vi "motors.vi"() -> (13 "Faults":bool[](array[boolean]), 14 "Left Drive 1":bool, 15 "Left Drive 2":bool, 16 "Left Drive 3":bool, 17 "Right Drive 1":bool, 18 "Right Drive 2":bool, 19 "Right Drive 3":bool)   [LabVIEW 2015]
uses:
  <vilib>/Rock Robotics/Network Tables/NT Read Number.vi
panel:
  out "Right Talon 1 Temperature Fault":i32
  out "Right Talon 1 Voltage Fault":i32
  out "Right Talon 1 Hardware Fault":i32
  out "Right Talon 2 Temperature Fault":i32
  out "Right Talon 2 Voltage Fault":i32
  out "Right Talon 2 Hardware Fault":i32
  out "Right Talon 3 Temperature Fault":i32
  out "Right Talon 3 Voltage Fault":i32
  out "Right Talon 3 Hardware Fault":i32
  out "Left Talon 3 Temperature Fault":i32
  out "Left Talon 3 Voltage Fault":i32
  out "Left Talon 3 Hardware Fault":i32
  out "Left Talon 2 Temperature Fault":i32
  out "Left Talon 2 Voltage Fault":i32
  out "Left Talon 2 Hardware Fault":i32
  out "Left Talon 1 Hardware Fault":i32
  out "Left Talon 1 Voltage Fault":i32
  out "Left Talon 1 Temperature Fault":i32
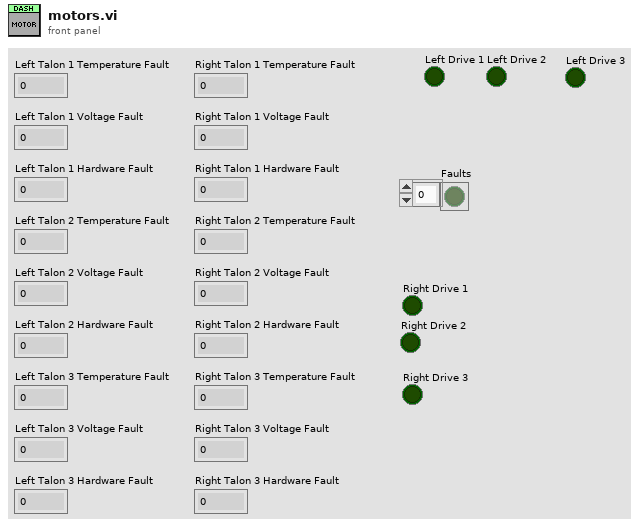
[diagram p1: front panel]
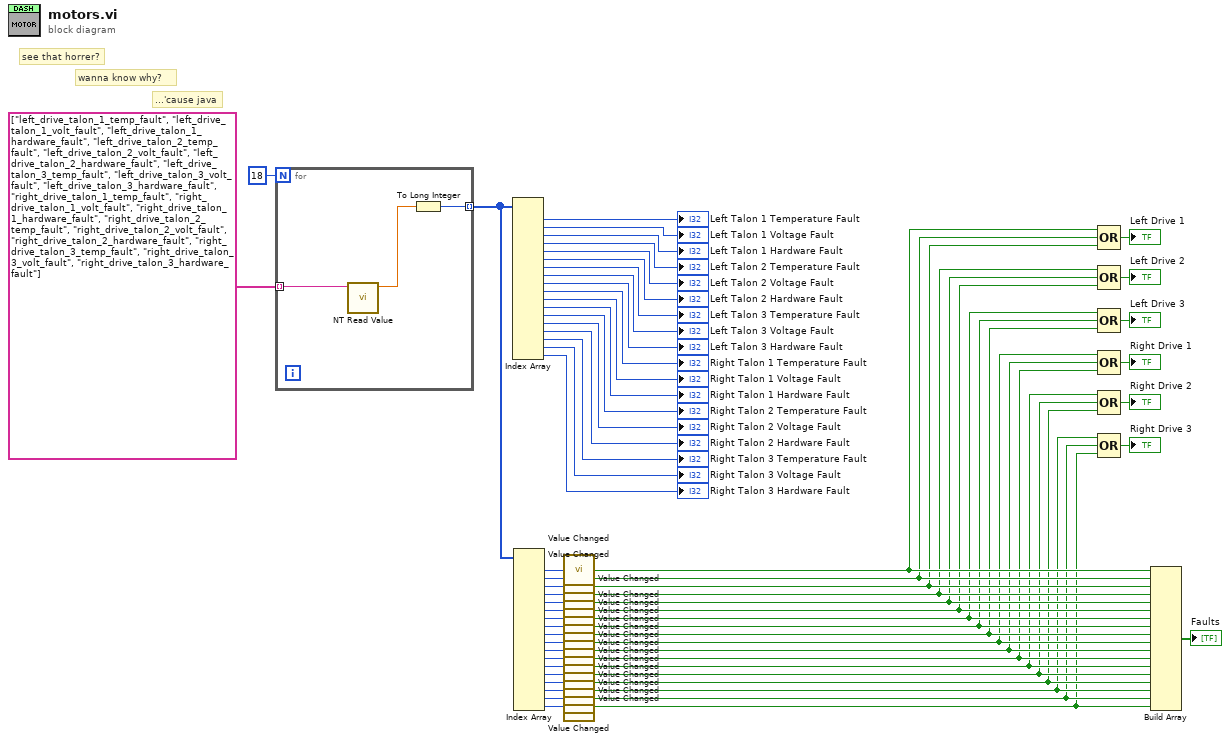
[diagram p0: block diagram]
diagram:
  # "wanna know why?"
  # "see that horrer?"
  # "...'cause java"
  n1 = for {
    N: 18 -> [_]
    tunnel: string[] ["left_drive_talon_1_temp_fault", "left_drive_talon_1_volt_fault", "left_drive_talon_1_hardware_fault", "left_drive_talon_2_temp_fault", "left_drive_talon_2_volt_fault", "left_drive_talon_2_hardware_fault", "left_drive_talon_3_temp_fault", "left_drive_talon_3_volt_fault", "left_drive_talon_3_hardware_fault", "right_drive_talon_1_temp_fault", "right_drive_talon_1_volt_fault", "right_drive_talon_1_hardware_fault", "right_drive_talon_2_temp_fault", "right_drive_talon_2_volt_fault", "right_drive_talon_2_hardware_fault", "right_drive_talon_3_temp_fault", "right_drive_talon_3_volt_fault", "right_drive_talon_3_hardware_fault"] -> [w67] mode=indexing
    tunnel: [w65] -> w44 mode=indexing
    n2 = call-poly <vilib>:"NT Read Value.vi"("Name"=w67) -> ("Numeric"=w66:dbl)  [unwired: 9 in, 1 out]
    n3 = To Long Integer(number=w66) -> (32bit integer=w65:i32)
  }
  n4 = Index Array(array=w44) -> (element #1=→"Left Talon 1 Temperature Fault":i32, element #2=→"Left Talon 1 Voltage Fault":i32, element #3=→"Left Talon 1 Hardware Fault":i32, element #4=→"Left Talon 2 Temperature Fault":i32, element #5=→"Left Talon 2 Voltage Fault":i32, element #6=→"Left Talon 2 Hardware Fault":i32, element #7=→"Left Talon 3 Temperature Fault":i32, element #8=→"Left Talon 3 Voltage Fault":i32, element #9=→"Left Talon 3 Hardware Fault":i32, element #10=→"Right Talon 1 Temperature Fault":i32, element #11=→"Right Talon 1 Voltage Fault":i32, element #12=→"Right Talon 1 Hardware Fault":i32, element #13=→"Right Talon 2 Temperature Fault":i32, element #14=→"Right Talon 2 Voltage Fault":i32, element #15=→"Right Talon 2 Hardware Fault":i32, element #16=→"Right Talon 3 Temperature Fault":i32, element #17=→"Right Talon 3 Voltage Fault":i32, element #18=→"Right Talon 3 Hardware Fault":i32)  [unwired: 18 in]
  n5 = Index Array(array=w44) -> (element #1=w43:i32, element #2=w42:i32, element #3=w41:i32, element #4=w40:i32, element #5=w39:i32, element #6=w38:i32, element #7=w37:i32, element #8=w36:i32, element #9=w35:i32, element #10=w34:i32, element #11=w33:i32, element #12=w32:i32, element #13=w31:i32, element #14=w30:i32, element #15=w29:i32, element #16=w28:i32, element #17=w27:i32, element #18=w26:i32)  [unwired: 18 in]
  n6 = call "Value Changed.vi"("Numeric"=w43) -> ("Changed"=w24:bool)  [unwired: 14 in]
  n7 = call "Value Changed.vi"("Numeric"=w42) -> ("Changed"=w23:bool)  [unwired: 14 in]
  n8 = call "Value Changed.vi"("Numeric"=w41) -> ("Changed"=w22:bool)  [unwired: 14 in]
  n9 = call "Value Changed.vi"("Numeric"=w40) -> ("Changed"=w21:bool)  [unwired: 14 in]
  n10 = call "Value Changed.vi"("Numeric"=w39) -> ("Changed"=w20:bool)  [unwired: 14 in]
  n11 = call "Value Changed.vi"("Numeric"=w38) -> ("Changed"=w19:bool)  [unwired: 14 in]
  n12 = call "Value Changed.vi"("Numeric"=w37) -> ("Changed"=w18:bool)  [unwired: 14 in]
  n13 = call "Value Changed.vi"("Numeric"=w36) -> ("Changed"=w17:bool)  [unwired: 14 in]
  n14 = call "Value Changed.vi"("Numeric"=w35) -> ("Changed"=w16:bool)  [unwired: 14 in]
  n15 = call "Value Changed.vi"("Numeric"=w34) -> ("Changed"=w15:bool)  [unwired: 14 in]
  n16 = call "Value Changed.vi"("Numeric"=w33) -> ("Changed"=w14:bool)  [unwired: 14 in]
  n17 = call "Value Changed.vi"("Numeric"=w32) -> ("Changed"=w13:bool)  [unwired: 14 in]
  n18 = call "Value Changed.vi"("Numeric"=w31) -> ("Changed"=w12:bool)  [unwired: 14 in]
  n19 = call "Value Changed.vi"("Numeric"=w30) -> ("Changed"=w11:bool)  [unwired: 14 in]
  n20 = call "Value Changed.vi"("Numeric"=w29) -> ("Changed"=w10:bool)  [unwired: 14 in]
  n21 = call "Value Changed.vi"("Numeric"=w28) -> ("Changed"=w9:bool)  [unwired: 14 in]
  n22 = call "Value Changed.vi"("Numeric"=w27) -> ("Changed"=w8:bool)  [unwired: 14 in]
  n23 = call "Value Changed.vi"("Numeric"=w26) -> ("Changed"=w7:bool)  [unwired: 14 in]
  n24 = Compound Arithmetic op=OR(w24, w23, w22) -> (→"Left Drive 1":bool)
  n25 = Compound Arithmetic op=OR(w21, w20, w19) -> (→"Left Drive 2":bool)
  n26 = Compound Arithmetic op=OR(w18, w17, w16) -> (→"Left Drive 3":bool)
  n27 = Compound Arithmetic op=OR(w15, w14, w13) -> (→"Right Drive 1":bool)
  n28 = Compound Arithmetic op=OR(w12, w11, w10) -> (→"Right Drive 2":bool)
  n29 = Compound Arithmetic op=OR(w9, w8, w7) -> (→"Right Drive 3":bool)
  n30 = Build Array(w24, w23, w22, w21, w20, w19, w18, w17, w16, w15, w14, w13, w12, w11, w10, w9, w8, w7) -> (→"Faults":bool[])
